vi "Find frame or struct.vi"(11 "GObj Refnum":refnum<vi>) -> (0 "error IO":errorcluster, 3 "cluster":T1)   [LabVIEW 2015]
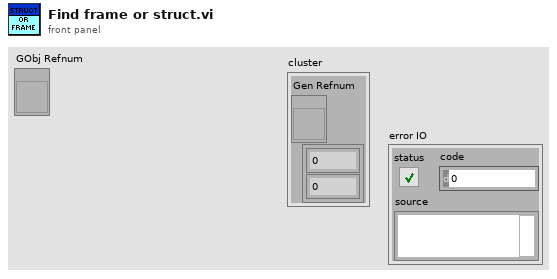
[diagram p1: front panel]
types:
  T1 = cluster{"Gen Refnum":refnum<vi>, "Postition":cluster{dbl, dbl}}
  T2 = typedef "LVBoundsTypeDef.ctl" = cluster{"Width":u32, "Height":u32}
  T3 = cluster{"Diagram.Owner":refnum<vi>, cluster{"Width":dbl, "Height":dbl}}
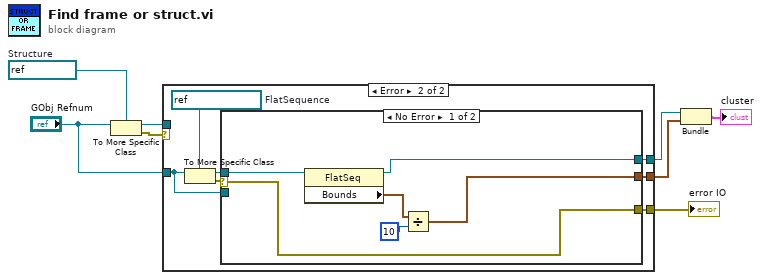
[diagram p0: block diagram]
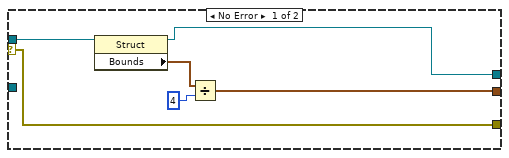
[diagram p2: hidden frame]
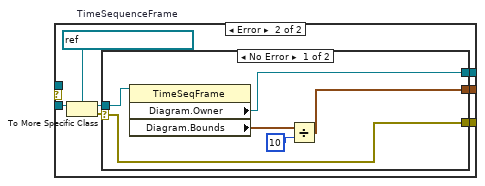
[diagram p3: hidden frame]
diagram:
  w7 = refnum<vi> refnum  # Structure
  n1 = To More Specific Class(target class=w7, reference="GObj Refnum") -> (specific class reference=w8:refnum<vi>, error out=w6:errorcluster)  [unwired: 1 in]
  n2 = case shown="Error" w6 {
    selector: w6 -> [w11 _]
    tunnel: w8 -> [w14 _]
    tunnel: "GObj Refnum" -> [_ w21]
    tunnel: [w10 w17] -> w4
    tunnel: [w11 w16] -> w5
    tunnel: [w9 w15] -> w2
    frame No Error {
      n3 = property class="Struct"(reference=w14) -> (reference out=w9:refnum<vi>, "Bounds"=w13:T2)  [unwired: 1 in, 1 out]
      n4 = Divide(x=w13, y=4) -> (x/y=w10:cluster{"Width":dbl, "Height":dbl})
    }
    frame Error {
      w18 = refnum<vi> refnum  # FlatSequence
      n5 = To More Specific Class(target class=w18, reference=w21) -> (specific class reference=w19:refnum<vi>, error out=w20:errorcluster)  [unwired: 1 in]
      n6 = case shown="No Error" w20 {
        selector: w20 -> [w24 _]
        tunnel: w21 -> [_ w34]
        tunnel: w19 -> [w25 _]
        tunnel: [w23 w30] -> w17
        tunnel: [w24 w29] -> w16
        tunnel: [w22 w28] -> w15
        frame No Error {
          n7 = property class="FlatSeq"(reference=w25) -> (reference out=w22:refnum<vi>, "Bounds"=w27:T2)  [unwired: 1 in, 1 out]
          n8 = Divide(x=w27, y=10) -> (x/y=w23:cluster{"Width":dbl, "Height":dbl})
        }
        frame Error {
          w33 = refnum<vi> refnum  # TimeSequenceFrame
          n9 = To More Specific Class(target class=w33, reference=w34) -> (specific class reference=w31:refnum<vi>, error out=w32:errorcluster)  [unwired: 1 in]
          n10 = case shown="No Error" w32 {
            selector: w32 -> [w37 w42]
            tunnel: w31 -> [w38 w41]
            tunnel: [w36 _] -> w30
            tunnel: [w37 w42] -> w29
            tunnel: [w35 w41] -> w28
            frame No Error {
              n11 = property class="TimeSeqFrame"(reference=w38) -> ("Diagram.Owner"=w35:refnum<vi>, "Diagram.Bounds"=w40:T2)  [unwired: 1 in, 2 out]
              n12 = Divide(x=w40, y=10) -> (x/y=w36:cluster{"Width":dbl, "Height":dbl})
            }
            frame Error {
            }
          }
        }
      }
    }
  }
  "error IO" <- w5
  n13 = Bundle("Diagram.Owner"=w2, w4) -> (→"cluster":T3)  [unwired: 1 in]
